vi "CSV_Setup_Data_Append_2.0.vi"(8 "Data":T1={"Camera 1"={"Camera1"="", "Cam 1"=FALSE, "CAM1 Model"=enum."a2A5328-15ucBAS", "Cam1 ID"=0}, "Camera 2"={"Camera2"="", "Cam 2"=FALSE, "CAM2 Model"=enum."a2A5328-15ucBAS", "Cam2 ID"=0}, "Image"={"Camera1_Img"=refnum, "Camera2_Img"=refnum, "Img1_Orig_Disp"=refnum, "Img2_Orig_Disp"=refnum, "Img1_Orig_RGB"=refnum, "Img2_Orig_RGB"=refnum, "Blue_Plane_Extract"=refnum, "Subtracted_Plane"=refnum, "Img1_Binary"=refnum, "Img2_Binary"=refnum, "Crop_Mask"=refnum, "Img1_Save"=refnum, "Img2_Save"=refnum, "Img1_Cali_Full"=refnum, "Img2_Cali_Full"=refnum, "Img1_Cali_Detect"=refnum, "Img2_Cali_Detect"=refnum}, "Ques"={"Cam 1 queue"=refnum, "Cam 2 queue"=refnum, "Cam 1 - save queue"=refnum, "Cam 2 - save queue"=refnum, "Image Process Queue Size"=500, "Image Save Queue Size"=500, "Overload threshold"=500, "Max large object threshold"=0}, "Arduino SRS"={"Pinch-valve"="", "Actuator"=FALSE, "Arduino Uno"="", "Valve state"=enum."Open"}, "Pump"={"Port"="", "Connection"=FALSE, "Flush Size"=0, "Command"="", "Pump Size"=enum."None", "Pump"="", "Ready"=FALSE}, "Camera settings"={"Detection settings"={"Sample size threshold"=500, "Detection Region %"=30.0, "Timeout Sample"=200}, "Lens/camera settings"={"Aperture"=enum."Item 0", "Legacy Cam Attributes"=FALSE, "Max Framerate"=100, "Exposure Time"=1000.0, "Framerate"=15}, "Crop settings"={"Cam1"={"Rectangle 1"={"Left"=0, "Top"=0, "Right"=0, "Bottom"=0, "Rotation"=0.0}, "Camera Orientation 1"="", "Pixel to mm 1"=0.0}, "Cam2"={"Rectangle 2"={"Left"=0, "Top"=0, "Right"=0, "Bottom"=0, "Rotation"=0.0}, "Camera Orientation 2"="", "Pixel to mm 2"=0.0}}}, "Arduino ISS"={"Mega F3"="", "Phase3"=FALSE, "Barcode"="", "Sorting sys."=FALSE, "Initial size"=0.0, "Size Interval"=0.0, "Mun. of containers"=0.0, "Container nr."=0.0, "Arduino Mega"="", "Attempts"=0.0}, "Img_Capt"=FALSE, "Empty_Refill"=FALSE, "I don't think is in use"={"Light intensity"=100}, "Extended setup"={"Location"="Station", "Latitude"="Station", "Longitude"="Station", "Determiner"="Station", "Sex"="Station", "Station"="", "Collection date"=""}, "Main interface"={"Sample Name"="Test Sample", "Operator"="JFR", "Species Name"="", "Other Notes"=""}, "Tap1"=0, "SystemVersion"=0, "System Serial"="", "Exit"=FALSE, "Kuvette Full"=FALSE, "Core JKI"={"Current VI Reference"=refnum, "Close Panel on Exit?"=FALSE}, "Calibration"={"Calibration 1"=path "C:/Users/au540322/Desktop/IHS_Project/images/Debris/Debris_0/Debris_0_2019_06_01-23-32-49-686.PNG", "Calibration 2"=path "C:/Users/au540322/Desktop/IHS_Project/images/Debris/Debris_0/Debris_0_2019_06_01-23-32-49-686.PNG", "Detect 1"=path "C:/Users/au540322/Desktop/IHS_Project/images/Debris/Debris_0/Debris_0_2019_06_01-23-32-49-686.PNG", "Detect 2"=path "C:/Users/au540322/Desktop/IHS_Project/images/Debris/Debris_0/Debris_0_2019_06_01-23-32-49-686.PNG"}, "Auto Flush"=FALSE, "Status History"="", "Timestamp Start"=""} {"SystemVersion" items=["Standard", "XL"]; "Tap1" items=["Session Data", "Extended Setup", "Buffer", "Camera", "Dispenser", "Stats", "Connections"]; "I don't think is in use"."Light intensity" scale=0.0..100.0; "Camera settings"."Crop settings"."Cam2"."Rectangle 2"."Rotation" format="%.2f"; "Camera settings"."Crop settings"."Cam2"."Rectangle 2"."Left" scale=0.0..1024.0; "Camera settings"."Crop settings"."Cam2"."Rectangle 2"."Right" scale=0.0..1024.0; "Camera settings"."Crop settings"."Cam1"."Rectangle 1"."Rotation" format="%.2f"; "Camera settings"."Crop settings"."Cam1"."Rectangle 1"."Left" scale=0.0..1024.0; "Camera settings"."Crop settings"."Cam1"."Rectangle 1"."Right" scale=0.0..1024.0; "Camera settings"."Lens/camera settings"."Framerate" min=1; "Camera settings"."Lens/camera settings"."Max Framerate" min=1; "Camera settings"."Detection settings"."Sample size threshold" min=1; "Pump"."Flush Size" min=0 max=6000 step=100; "Ques"."Overload threshold" min=1; "Ques"."Image Save Queue Size" min=1; "Ques"."Image Process Queue Size" min=1}, 9 "Sample cluster":T5, 10 "Sample Name":string, 11 "Image path":string) -> (2 "File Path":string, 3 "Sample Name dup":string)   [LabVIEW 2024]
uses:
  controls/Data_JKI.ctl
  <vilib>/userDefined/High Color/IMAQdx.ctl
  <vilib>/vision/Image Controls.llb/IMAQ Image.ctl
  <vilib>/Utility/file.llb/Write Delimited Spreadsheet (string).vi
panel:
  out "string":string
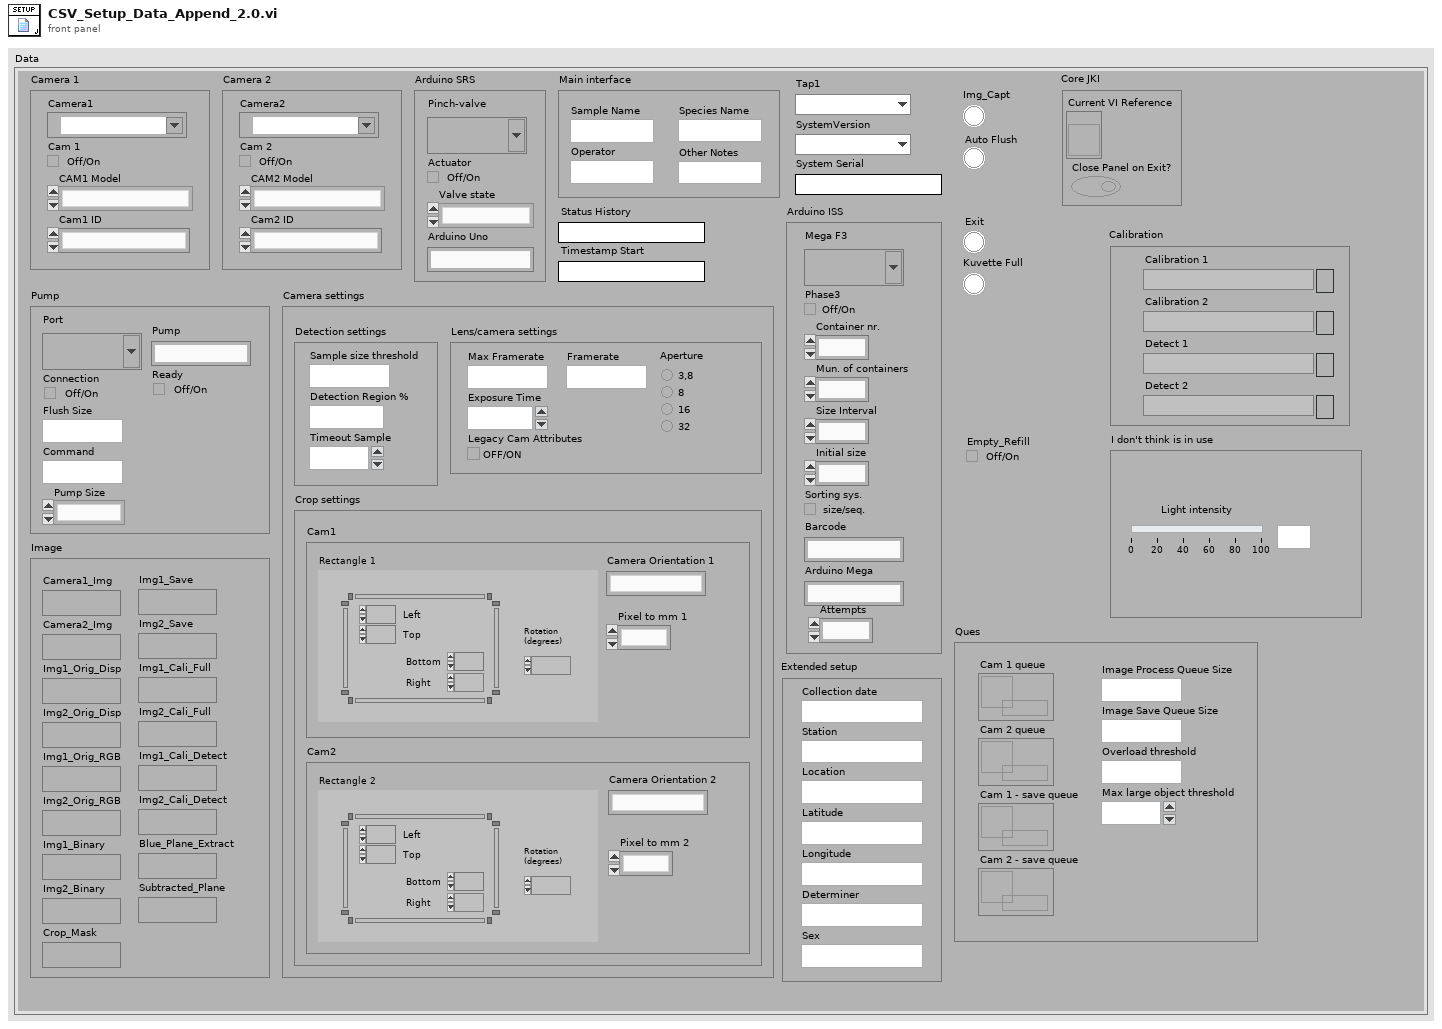
[diagram p1: front panel]
types:
  T1 = typedef "Data_JKI.ctl" = cluster{"Camera 1":cluster{"Camera1":T2, "Cam 1":bool, "CAM1 Model":enum16{"a2A5328-15ucBAS", "acA1920-155uc"}, "Cam1 ID":i32}, "Camera 2":cluster{"Camera2":T2, "Cam 2":bool, "CAM2 Model":enum16{"a2A5328-15ucBAS", "acA1920-155uc"}, "Cam2 ID":i32}, "Image":cluster{"Camera1_Img":T3, "Camera2_Img":T3, "Img1_Orig_Disp":T3, "Img2_Orig_Disp":T3, "Img1_Orig_RGB":T3, "Img2_Orig_RGB":T3, "Blue_Plane_Extract":T3, "Subtracted_Plane":T3, "Img1_Binary":T3, "Img2_Binary":T3, "Crop_Mask":T3, "Img1_Save":T3, "Img2_Save":T3, "Img1_Cali_Full":T3, "Img2_Cali_Full":T3, "Img1_Cali_Detect":T3, "Img2_Cali_Detect":T3}, "Ques":cluster{"Cam 1 queue":refnum<queue>, "Cam 2 queue":refnum<queue>, "Cam 1 - save queue":refnum<queue>, "Cam 2 - save queue":refnum<queue>, "Image Process Queue Size":i32, "Image Save Queue Size":i32, "Overload threshold":i32, "Max large object threshold":i32}, "Arduino SRS":cluster{"Pinch-valve":refnum<visa-resource-name>, "Actuator":bool, "Arduino Uno":string, "Valve state":enum16{"Standby", "Close", "Open"}}, "Pump":cluster{"Port":refnum<visa-resource-name>, "Connection":bool, "Flush Size":i32, "Command":string, "Pump Size":enum16{"None", "Small", "Large"}, "Pump":string, "Ready":bool}, "Camera settings":cluster{"Detection settings":cluster{"Sample size threshold":i32, "Detection Region %":dbl, "Timeout Sample":i32}, "Lens/camera settings":cluster{"Aperture":enum32{"Item 0", "Item 1", "Item 2", "Item 3"}, "Legacy Cam Attributes":bool, "Max Framerate":i32, "Exposure Time":dbl, "Framerate":i32}, "Crop settings":cluster{"Cam1":cluster{"Rectangle 1":T4, "Camera Orientation 1":string, "Pixel to mm 1":dbl}, "Cam2":cluster{"Rectangle 2":T4, "Camera Orientation 2":string, "Pixel to mm 2":dbl}}}, "Arduino ISS":cluster{"Mega F3":refnum<visa-resource-name>, "Phase3":bool, "Barcode":string, "Sorting sys.":bool, "Initial size":dbl, "Size Interval":dbl, "Mun. of containers":dbl, "Container nr.":dbl, "Arduino Mega":string, "Attempts":dbl}, "Img_Capt":bool, "Empty_Refill":bool, "I don't think is in use":cluster{"Light intensity":i32}, "Extended setup":cluster{"Location":string, "Latitude":string, "Longitude":string, "Determiner":string, "Sex":string, "Station":string, "Collection date":string}, "Main interface":cluster{"Sample Name":string, "Operator":string, "Species Name":string, "Other Notes":string}, "Tap1":u16, "SystemVersion":u16, "System Serial":string, "Exit":bool, "Kuvette Full":bool, "Core JKI":cluster{"Current VI Reference":refnum<vi>, "Close Panel on Exit?":bool}, "Calibration":cluster{"Calibration 1":path, "Calibration 2":path, "Detect 1":path, "Detect 2":path}, "Auto Flush":bool, "Status History":string, "Timestamp Start":string}
  T2 = typedef "IMAQdx.ctl" = refnum<k21>
  T3 = typedef "IMAQ Image.ctl" = refnum<image>
  T4 = typedef "IMAQ Rectangle" = cluster{"Left":i32, "Top":i32, "Right":i32, "Bottom":i32, "Rotation":dbl}
  T5 = cluster{"MFD max":string, "MFD mean":string, "MFD std. dev.":string, "Perim. mean":string, "Perim. std. dev":string, "Area mean":string, "Area std. dev.":string, "Holes mean":string, "Holes std. dev.":string, "Area+Holes mean":string, "Area+Holes std. dev.":string, "Container barcode":string}
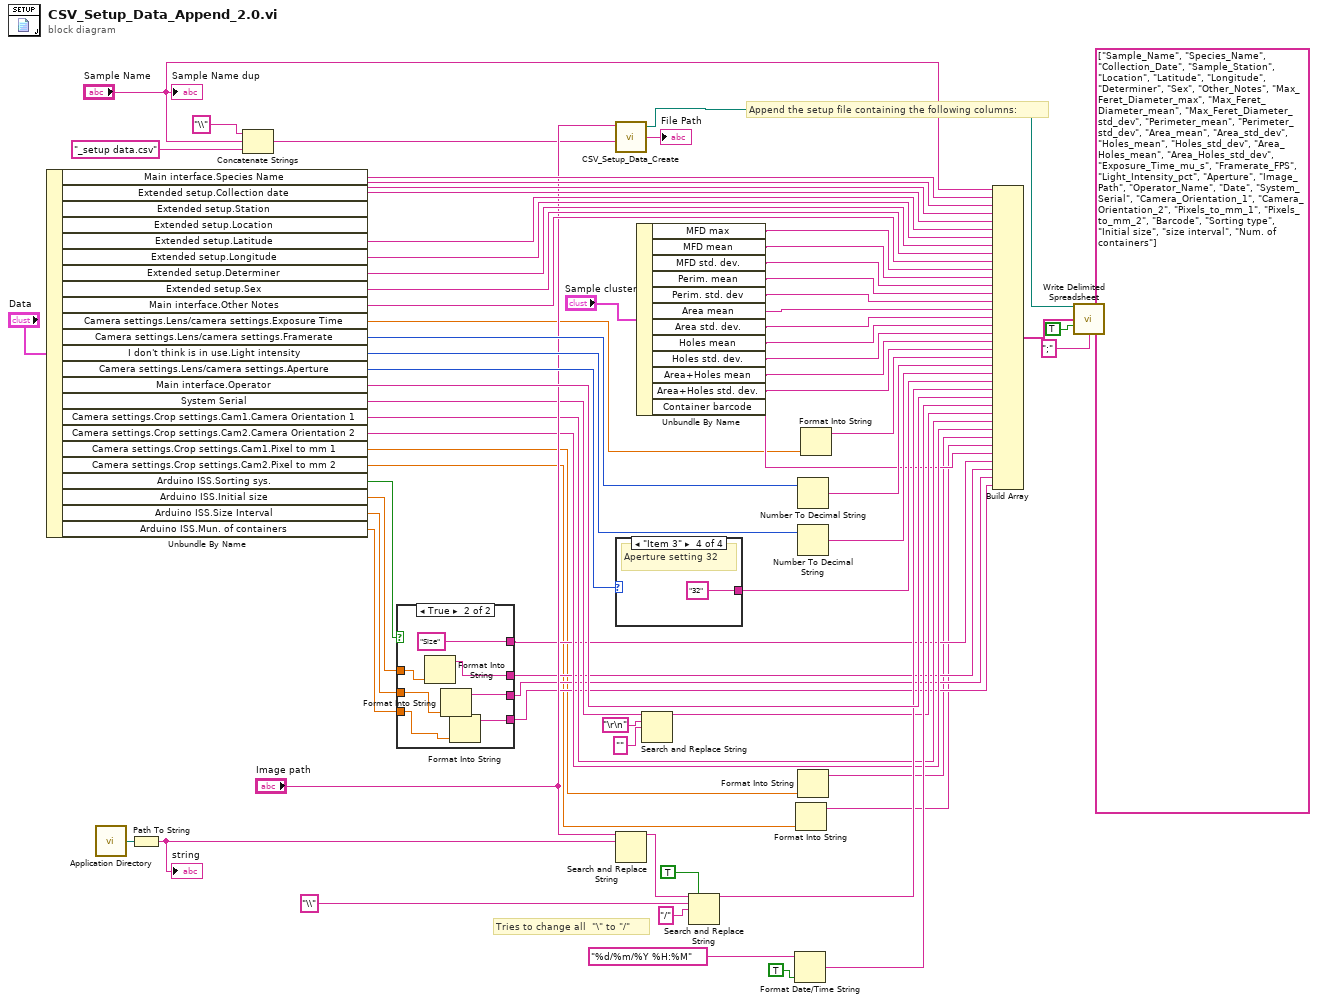
[diagram p0: block diagram]
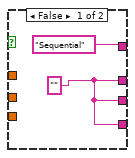
[diagram p2: hidden frame]
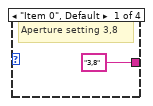
[diagram p3: hidden frame]
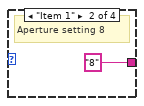
[diagram p4: hidden frame]
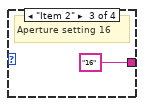
[diagram p5: hidden frame]
diagram:
  (unwired) string[] ["Sample_Name", "Species_Name", "Collection_Date", "Sample_Station", "Location", "Latitude", "Longitude", "Determiner", "Sex", "Other_Notes", "Max_Feret_Diameter_max", "Max_Feret_Diameter_mean", "Max_Feret_Diameter_std_dev", "Perimeter_mean", "Perimeter_std_dev", "Area_mean", "Area_std_dev", "Holes_mean", "Holes_std_dev", "Area_Holes_mean", "Area_Holes_std_dev", "Exposure_Time_mu_s", "Framerate_FPS", "Light_Intensity_pct", "Aperture", "Image_Path", "Operator_Name", "Date", "System_Serial", "Camera_Orientation_1", "Camera_Orientation_2", "Pixels_to_mm_1", "Pixels_to_mm_2", "Barcode", "Sorting type", "Initial size", "size interval", "Num. of containers"]
  # "Tries to change all  \"\\\" to \"/\""
  # "Append the setup file containing the following columns:"
  n1 = Unbundle By Name("Data") -> ("Main interface.Species Name"=w49:string, "Extended setup.Collection date"=w50:string, "Extended setup.Station"=w51:string, "Extended setup.Location"=w52:string, "Extended setup.Latitude"=w53:string, "Extended setup.Longitude"=w54:string, "Extended setup.Determiner"=w55:string, "Extended setup.Sex"=w56:string, "Main interface.Other Notes"=w57:string, "Camera settings.Lens/camera settings.Exposure Time"=w2:dbl, "Camera settings.Lens/camera settings.Framerate"=w65:i32, "I don't think is in use.Light intensity"=w64:i32, "Camera settings.Lens/camera settings.Aperture"=w63:enum32{"Item 0", "Item 1", "Item 2", "Item 3"}, "Main interface.Operator"=w59:string, "System Serial"=w33:string, "Camera settings.Crop settings.Cam1.Camera Orientation 1"=w35:string, "Camera settings.Crop settings.Cam2.Camera Orientation 2"=w34:string, "Camera settings.Crop settings.Cam1.Pixel to mm 1"=w6:dbl, "Camera settings.Crop settings.Cam2.Pixel to mm 2"=w5:dbl, "Arduino ISS.Sorting sys."=w14:bool, "Arduino ISS.Initial size"=w13:dbl, "Arduino ISS.Size Interval"=w12:dbl, "Arduino ISS.Mun. of containers"=w11:dbl)
  n2 = call <vilib>:"Application Directory.vi"() -> ("Application Directory"=w67:path)
  n3 = Path To String(path=w67) -> (string=w66:string)
  "string" <- w66
  n4 = Concatenate Strings("\\" ("string"), "Sample Name", "_setup data.csv") -> (w43:string)
  n5 = case shown="True" w14 {
    tunnel: w13 -> [_ w76]
    tunnel: w12 -> [_ w77]
    tunnel: w11 -> [_ w78]
    tunnel: [w71 w73] -> w7
    tunnel: [w71 w74] -> w8
    tunnel: [w71 w75] -> w9
    tunnel: ["Sequential" "Size"] -> w10
    frame False {
      w71 = ""
    }
    frame True {
      n6 = Format Into String(w76) -> (resulting string=w75:string)  [unwired: 3 in, 1 out]
      n7 = Format Into String(w77) -> (resulting string=w74:string)  [unwired: 3 in, 1 out]
      n8 = Format Into String(w78) -> (resulting string=w73:string)  [unwired: 3 in, 1 out]
    }
  }
  n9 = call "CSV_Setup_Data_Create.vi"("Setup Data File"=w43, "Setup Data path"="Image path") -> ("File Path"=→"File Path":string, "Setup Data File path"=w45:path)  [unwired: 2 in, 1 out]
  n10 = case shown="\"Item 3\"" w63 {
    tunnel: ["3,8" "8" "16" "32"] -> w60
    frame "Item 0", Default {
      # "Aperture setting 3,8"
    }
    frame "Item 1" {
      # "Aperture setting 8"
    }
    frame "Item 2" {
      # "Aperture setting 16"
    }
    frame "Item 3" {
      # "Aperture setting 32"
    }
  }
  n11 = Search and Replace String(input string="Image path", search string=w66) -> (result string=w37:string)  [unwired: 6 in, 3 out]
  n12 = Unbundle By Name("Sample cluster") -> ("MFD max"=w27:string, "MFD mean"=w26:string, "MFD std. dev."=w25:string, "Perim. mean"=w24:string, "Perim. std. dev"=w23:string, "Area mean"=w22:string, "Area std. dev."=w21:string, "Holes mean"=w20:string, "Holes std. dev."=w19:string, "Area+Holes mean"=w18:string, "Area+Holes std. dev."=w17:string, "Container barcode"=w16:string)
  n13 = Search and Replace String(input string=w33, search string="\r\n", replace string="" ("replace string (\"\")")) -> (result string=w32:string)  [unwired: 5 in, 3 out]
  n14 = Search and Replace String(replace all?=TRUE ("replace all? (F)"), input string=w37, search string="\\", replace string="/" ("replace string (\"\")")) -> (result string=w36:string)  [unwired: 4 in, 3 out]
  n15 = Format Date/Time String(time format string (%c)="%d/%m/%Y %H:%M", UTC format=TRUE) -> (date/time string=w58:string)  [unwired: 1 in]
  n16 = Format Into String(w5) -> (resulting string=w4:string)  [unwired: 3 in, 1 out]
  n17 = Number To Decimal String(number=w65) -> (decimal integer string=w62:string)  [unwired: 1 in]
  n18 = Number To Decimal String(number=w64) -> (decimal integer string=w61:string)  [unwired: 1 in]
  n19 = Format Into String(w6) -> (resulting string=w3:string)  [unwired: 3 in, 1 out]
  n20 = Format Into String(w2) -> (resulting string=w1:string)  [unwired: 3 in, 1 out]
  n21 = Build Array("Sample Name", w49, w50, w51, w52, w53, w54, w55, w56, w57, w27, w26, w25, w24, w23, w22, w21, w20, w19, w18, w17, w1, w62, w61, w60, w36, w59, w58, w32, w35, w34, w3, w4, w16, w10, w9, w8, w7) -> (w29:string[])
  n22 = call-poly <vilib>:"Write Delimited Spreadsheet.vi"("file path (dialog if empty)"=w45, "1D data"=w29, "append to file? (new file:F)"=TRUE, "delimiter (\\t)"=";" ("delimiter (\\t)")) -> ()  [unwired: 10 in, 2 out]
  "Sample Name dup" <- "Sample Name"
